vi "UiControls_gas.vi"() -> ()   [LabVIEW 2011]
uses:
  Output - Cluster gas.ctl
  Input - Cluster gas.ctl
panel:
  out "measuring mode 2":u8
  in  "measuring volume":u32
  in  "Tab Control":enum32{"controls", "tools"}(tab)
  in  "measuring point":u32(ring) items=["-"=0, "Fabes 2 MR"=1, "Fabes 2 HR"=2, "Fabes 1 MR"=4, "Fabes 1 BL"=8, "Fabes 1 HR"=16, "B2G 1 HR"=32, "B2G 1 T-2"=64, "B2G 1 MR"=128, "B2G 2 T-2"=256, "B2G 2 MR"=512]
  in  "measuring mode":u8(ring) items=["quality & quantity"=3, "quality"=1, "quantity"=2, "-"=0, "flushing"=9]
  in  "start":bool
  in  "dosage timetable":bool caption="activate"
  in  "Zeitplan":string[][](table)=[["00:00", "0", "1", "1", "1,5"], ["01:00", "0", "1", "1", "1,5"], ["02:00", "0", "1", "1", "1,5"], ["03:00", "0", "1", "1", "1,5"], ["04:00", "0", "1", "1", "1,5"], ["05:00", "0", "1", "1", "1,5"], ["06:00", "0", "1", "1", "1,5"], ["07:00", "0", "1", "1", "1,5"], ["08:00", "0", "1", "1", "1,5"], ["09:00", "0", "1", "1", "1,5"], ["10:00", "0", "1", "1", "1,5"], ["11:00", "0", "1", "1", "1,5"], ["12:00", "0", "1", "1", "1,5"], ["13:00", "0", "1", "1", "1,5"], ["14:00", "0", "1", "1", "1,5"], ["15:00", "0", "1", "1", "1,5"], ["16:00", "0", "1", "1", "1,5"], ["17:00", "0", "1", "1", "1,5"], ["18:00", "0", "1", "1", "1,5"], ["19:00", "0", "1", "1", "1,5"], ["20:00", "0", "1", "1", "1,5"], ["21:00", "0", "1", "1", "1,5"], ["22:00", "0", "1", "1", "1,5"], ["23:00", "0", "1", "1", "1,5"]]
  in  "stop":bool caption="stop crio"
  out "pc":timestamp
  out "crio":timestamp
  in  "load/save":enum16{"Load", "Save"}(ring)
  in  "enter":bool
  in  "config file":path caption="path"
  in  "crio log":bool
  out "status":string
  # "timestamp"
  # "configurtaion file"
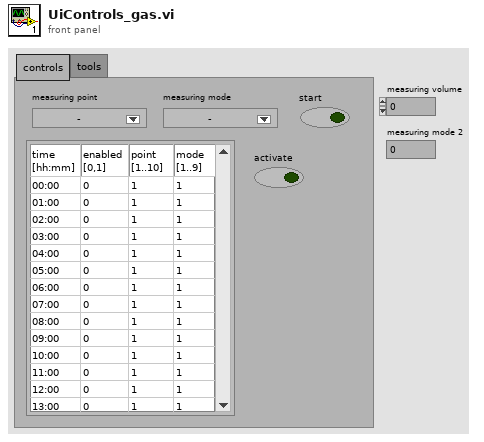
[diagram p1: front panel]
types:
  T1 = typedef "Output - Cluster gas.ctl" = cluster{"B2G2 MR V1.1 AUF":bool, "B2G2 MR V1.1 ZU":bool, "B2G2 MR V1 AUF":bool, "B2G2 MR V1 ZU":bool, "B2G1 T2 V1 AUF":bool, "B2G1 T2 V1 ZU":bool, "B2G1 T2 V1.1 AUF":bool, "B2G1 T2 V1.1 ZU":bool, "B2G2 T2 V1 AUF":bool, "B2G2 T2 V1 ZU":bool, "B2G2 T2 V1.1 ZU":bool, "B2G2 T2 V1.1 AUF":bool, "B2G1 MR V1 AUF":bool, "B2G1 MR V1 ZU":bool, "B2G1 MR V1.1 AUF":bool, "B2G1 MR V1.1 ZU":bool, "B2G1 HR V1 AUF":bool, "B2G1 HR V1 ZU":bool, "B2G1 HR V1.1 AUF":bool, "B2G1 HR V1.1 ZU":bool, "Fab1 HR V1 AUF":bool, "Fab1 HR V1 ZU":bool, "Fab1 HR V1.1 AUF":bool, "Fab1 HR V1.1 ZU":bool, "Fab1 MR V1 AUF":bool, "Fab1 MR V1 ZU":bool, "Fab1 MR V1.1 AUF":bool, "Fab1 MR V1.1 ZU":bool, "Fab1 BL V1 AUF":bool, "Fab1 BL V1 ZU":bool, "Fab1 BL V1.1 AUF":bool, "Fab1 BL V1.1 ZU":bool, "Fab2 HR V1 AUF":bool, "Fab2 HR V1 ZU":bool, "Fab2 HR V1.1 AUF":bool, "Fab2 HR V1.1 ZU":bool, "Fab2 MR V1 AUF":bool, "Fab2 MR V1 ZU":bool, "Fab2 MR V1.1 AUF":bool, "Fab2 MR V1.1 ZU":bool, "GA1 ch4 [%]":dbl, "GA1 co2 [%]":dbl, "GA1 h2 [%]":dbl, "GM P1 RUN":bool, "GM V-1 AUF":bool, "GM V-1 ZU":bool, "GM V-2 AUF":bool, "GM V-2 ZU":bool, "GM V-3 AUF":bool, "GM V-3 ZU":bool, "GM V-4 AUF":bool, "GM V-4 ZU":bool, "GM P2 RUN":bool, "GM GZ-1 [imp]":u32, "GM DS-2 [bar]":dbl, "GM DS-1 [bar]":dbl, "GM TS-1 [°C]":dbl, "GM TS-2[°C]":dbl, "gas_values":cluster{"timestamp":timestamp, "GM DS-2 [bar]":dbl, "GA1 ch4 [%]":dbl, "GA1 co2 [%]":dbl, "GA1 h2 [%]":dbl, "GM DS-1 [bar]":dbl, "GM TS-1 [°C]":dbl, "GM TS-2 [°C]":dbl, "GM GZ-1 [l]":dbl, "empty":bool, "measuring point":u8}, "measuring mode":u8}
  T2 = typedef "Input - Cluster gas.ctl" = cluster{"GM P-1":bool, "GM P-2":bool, "measuring point":u32, "measuring mode":u8, "GM-V1,2":bool, "GM-V3,4":bool, "GM-V5":bool, "measuring volume":u32}
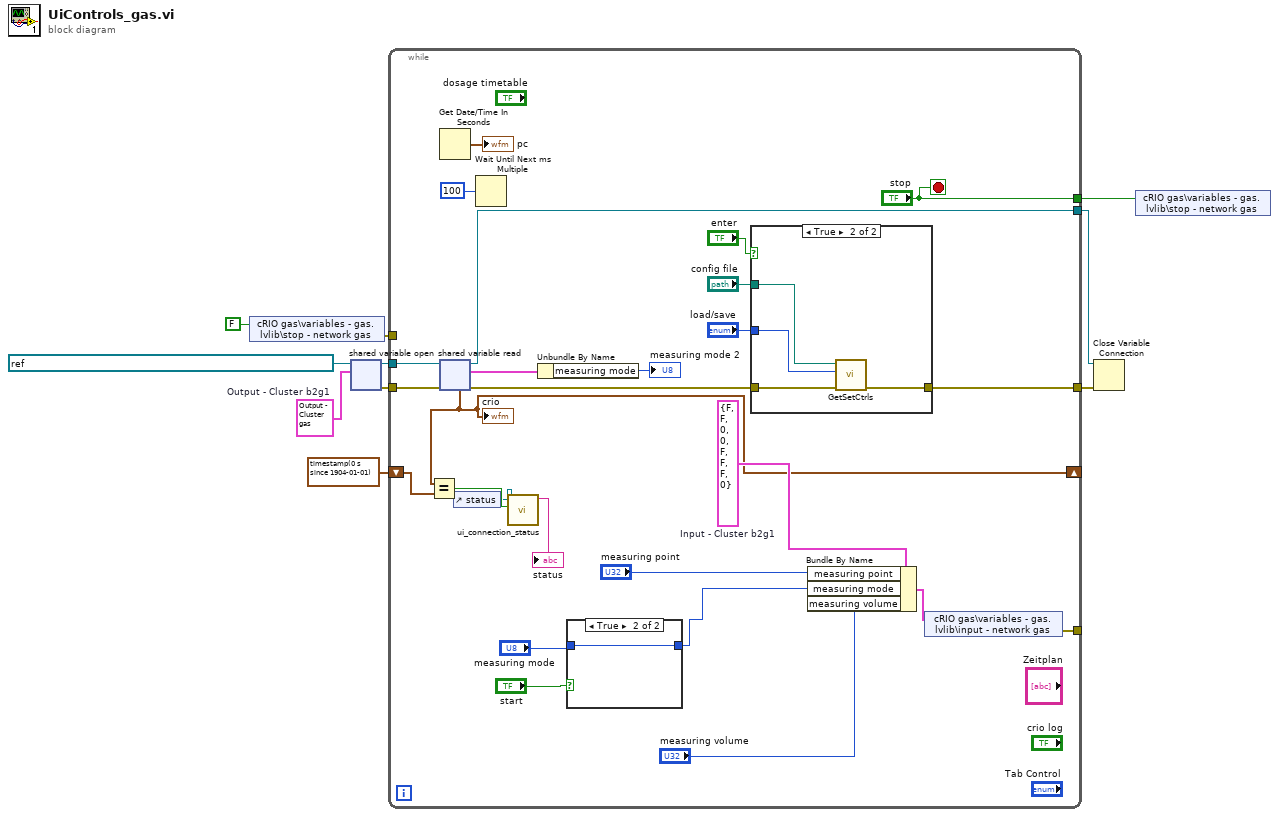
[diagram p0: block diagram]
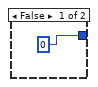
[diagram p2: hidden frame]
diagram:
  w2 = T1 {"B2G2 MR V1.1 AUF"=FALSE, "B2G2 MR V1.1 ZU"=FALSE, "B2G2 MR V1 AUF"=FALSE, "B2G2 MR V1 ZU"=FALSE, "B2G1 T2 V1 AUF"=FALSE, "B2G1 T2 V1 ZU"=FALSE, "B2G1 T2 V1.1 AUF"=FALSE, "B2G1 T2 V1.1 ZU"=FALSE, "B2G2 T2 V1 AUF"=FALSE, "B2G2 T2 V1 ZU"=FALSE, "B2G2 T2 V1.1 ZU"=FALSE, "B2G2 T2 V1.1 AUF"=FALSE, "B2G1 MR V1 AUF"=FALSE, "B2G1 MR V1 ZU"=FALSE, "B2G1 MR V1.1 AUF"=FALSE, "B2G1 MR V1.1 ZU"=FALSE, "B2G1 HR V1 AUF"=FALSE, "B2G1 HR V1 ZU"=FALSE, "B2G1 HR V1.1 AUF"=FALSE, "B2G1 HR V1.1 ZU"=FALSE, "Fab1 HR V1 AUF"=FALSE, "Fab1 HR V1 ZU"=FALSE, "Fab1 HR V1.1 AUF"=FALSE, "Fab1 HR V1.1 ZU"=FALSE, "Fab1 MR V1 AUF"=FALSE, "Fab1 MR V1 ZU"=FALSE, "Fab1 MR V1.1 AUF"=FALSE, "Fab1 MR V1.1 ZU"=FALSE, "Fab1 BL V1 AUF"=FALSE, "Fab1 BL V1 ZU"=FALSE, "Fab1 BL V1.1 AUF"=FALSE, "Fab1 BL V1.1 ZU"=FALSE, "Fab2 HR V1 AUF"=FALSE, "Fab2 HR V1 ZU"=FALSE, "Fab2 HR V1.1 AUF"=FALSE, "Fab2 HR V1.1 ZU"=FALSE, "Fab2 MR V1 AUF"=FALSE, "Fab2 MR V1 ZU"=FALSE, "Fab2 MR V1.1 AUF"=FALSE, "Fab2 MR V1.1 ZU"=FALSE, "GA1 ch4 [%]"=0.0, "GA1 co2 [%]"=0.0, "GA1 h2 [%]"=0.0, "GM P1 RUN"=FALSE, "GM V-1 AUF"=FALSE, "GM V-1 ZU"=FALSE, "GM V-2 AUF"=FALSE, "GM V-2 ZU"=FALSE, "GM V-3 AUF"=FALSE, "GM V-3 ZU"=FALSE, "GM V-4 AUF"=FALSE, "GM V-4 ZU"=FALSE, "GM P2 RUN"=FALSE, "GM GZ-1 [imp]"=0, "GM DS-2 [bar]"=0.0, "GM DS-1 [bar]"=0.0, "GM TS-1 [°C]"=0.0, "GM TS-2[°C]"=0.0, "gas_values"={"timestamp"=timestamp(0 s since 1904-01-01), "GM DS-2 [bar]"=0.0, "GA1 ch4 [%]"=0.0, "GA1 co2 [%]"=0.0, "GA1 h2 [%]"=0.0, "GM DS-1 [bar]"=0.0, "GM TS-1 [°C]"=0.0, "GM TS-2 [°C]"=0.0, "GM GZ-1 [l]"=0.0, "empty"=FALSE, "measuring point"=0}, "measuring mode"=0}  # Output - Cluster b2g1
  n1 = shared-variable "cRIO gas\\variables - gas.lvlib\\stop - network gas"(FALSE ("stop - network")) -> (error out=w9:errorcluster)  [unwired: 1 in]
  n2 = shared-variable-open(refnum<k21> "ni.var.psp://10.27.40.21/variables - gas/data - network - gas" ("shared variable refnum in"), w2) -> (w6:refnum<k21>, w4:errorcluster)  [unwired: 2 in]
  n3 = while {
    tunnel: ["stop"] -> w10
    tunnel: w9 -> [_]
    tunnel: [w34] -> _
    tunnel: w6 -> [w31]
    tunnel: [w29] -> w5
    tunnel: w4 -> [w28]
    tunnel: [w24] -> w3
    shift-right: [w11] -> _
    shift-left: timestamp(0 s since 1904-01-01) -> [w12]
    stop <- "stop" stop-if-true
    w36 = T2 {"GM P-1"=FALSE, "GM P-2"=FALSE, "measuring point"=0, "measuring mode"=0, "GM-V1,2"=FALSE, "GM-V3,4"=FALSE, "GM-V5"=FALSE, "measuring volume"=0}  # Input - Cluster b2g1
    n4 = Get Date/Time In Seconds() -> (seconds since 1Jan1904=→"pc":timestamp)
    n5 = shared-variable-read(w31, w28) -> (w29:refnum<k21>, w25:errorcluster, w30:T1, w11:timestamp)
    "crio" <- w11
    n6 = Equal?(x=w11, y=w12) -> (x = y?=w15:bool)
    n7 = control-ref of="status"() -> (w14:refnum<vi>)
    n8 = Wait Until Next ms Multiple(millisecond multiple=u32 100) -> ()  [unwired: 1 out]
    n9 = call "ui_connection_status.vi"("Boolean"=w15, "String in"=w14) -> ("status"=→"status":string)  [unwired: 9 in]
    n10 = Unbundle By Name(w30) -> ("measuring mode"=→"measuring mode 2":u8)
    n11 = case shown="True" "start" {
      tunnel: [u8 0 ("measuring point") w38] -> w18
      tunnel: "measuring mode" -> [_ w38]
      frame False {
      }
      frame True {
      }
    }
    n12 = case shown="True" "enter" {
      tunnel: w25 -> [w39 w43]
      tunnel: [w39 w42] -> w24
      tunnel: "load/save" -> [_ w41]
      tunnel: "config file" -> [_ w40]
      frame False {
      }
      frame True {
        n13 = call "GetSetCtrls.vi"("error in (no error)"=w43, "Function (Load)"=w41, "Ini file (empty)"=w40) -> ("error out"=w42:errorcluster)  [unwired: 8 in]
      }
    }
    n14 = Bundle By Name(cluster=w36, "measuring point"="measuring point", "measuring mode"=w18, "measuring volume"="measuring volume") -> (w35:T2)
    n15 = shared-variable "cRIO gas\\variables - gas.lvlib\\input - network gas"(w35) -> (error out=w34:errorcluster)  [unwired: 1 in]
  }
  n16 = Close Variable Connection(8:w3, 11:w5) -> ()  [unwired: 1 out]
  n17 = shared-variable "cRIO gas\\variables - gas.lvlib\\stop - network gas"(w10) -> ()  [unwired: 1 in, 1 out]
